vi "Enqueue.vi"(8 "error in (no error)":errorcluster, 9 "Data":variant, 10 "Action":T1, 11 "Subsystem":T2=enum."SonicShifter") -> (0 "error out":errorcluster)   [LabVIEW 2013]
uses:
  QueueSubsystem.ctl
  QueueAction.ctl
  QueueInstruction.ctl
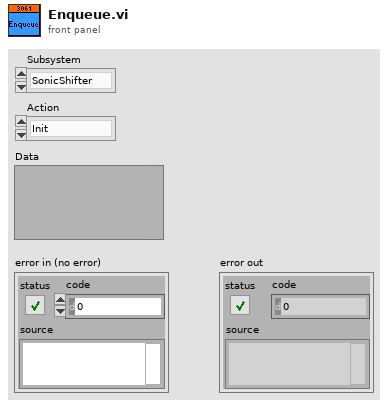
[diagram p1: front panel]
types:
  T1 = typedef "QueueAction.ctl" = enum16{"Init", "SetValue", "Disable"}
  T2 = typedef "QueueSubsystem.ctl" = enum16{"Drive", "SonicShifter", "Kicker", "FiringPneumatic", "RollerPneumatic", "Clapper", "RollerMotor", "CollectorMotor", "PressureSensor", "Servo", "ShooterWrapper", "CollectorWrapper", "CatcherWrapper", "AutoDistance", "PassWrapper"}
  T3 = typedef "QueueInstruction.ctl" = cluster{"Data":variant, "Subsystem":T2, "Action":T1}
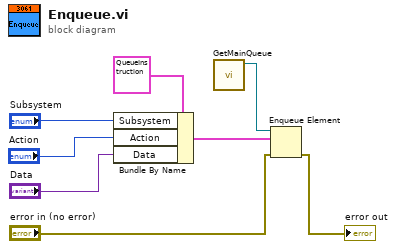
[diagram p0: block diagram]
diagram:
  n1 = Bundle By Name(cluster=T3 {"Data"=variant, "Subsystem"=enum."SonicShifter", "Action"=enum."Init"} ("QueueInstruction"), "Subsystem"="Subsystem", "Action"="Action", "Data"="Data") -> (w3:T3)
  n2 = call "GetMainQueue.vi"() -> ("queue out"=w4:refnum<queue>)  [unwired: 10 in, 1 out]
  n3 = Enqueue Element(queue=w4, element=w3, error in (no error)="error in (no error)") -> (error out=→"error out":errorcluster)  [unwired: 1 in, 2 out]
